vi "Draw Current Position Marker.vi"(8 "Error":errorcluster, 9 "Waveform":waveform(dbl), 10 "State":T1={"Measure ?"=[], "Direction"=[], "Loop ?"={"Start"=0, "Finish"=2}, "Storage Location"=[], "Show Current Location"=FALSE, "Current Location"=0, "Show y=0"=FALSE, "Program"=[], "Index"=0, "Average During Loop ?"=FALSE, "# of Loops"=1, "Loop Control"={0, 2}, "Units"="", "Digits"=0, "Significant Figures (F) or DP (T)"=FALSE, "Rate Mode"=FALSE, "Current Y value"=0.0, "Initial Value"=0.0} {"# of Loops" min=1 step=1; "Index" min=0 step=1; "Program"."Step" min=0.001 max=80.0 step=0.001 format="%.2f"; "Program"."Target" format="%.2f"}, 11 "Plots":cluster{"X":dbl[], "Y":dbl[]}[](array[cluster])) -> (0 "Error Out":errorcluster, 3 "Plots Out":cluster{"X":dbl[], "Y":dbl[]}[](array[cluster]))   [LabVIEW 2018, in "Multi Segment Waveform.xctl"]
doc: "Generates a waveform that is NaN apart from the one point at the given index position. The Y value of this point is the same as the corresponding point in the first waveform of the array input,"
uses:
  Multi Segment Waveform.xctl
  State.ctl
  <vilib>/Waveform/WDTOps.llb/WDT Get XY Value DBL.vi
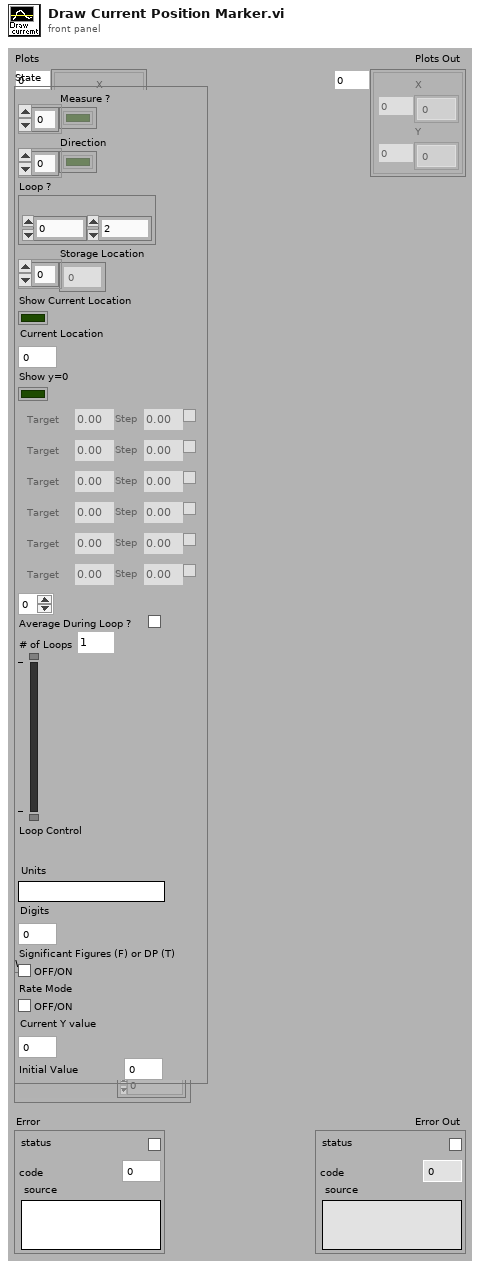
[diagram p1: front panel]
types:
  T1 = typedef "Multi Segment Waveform.xctl/State.ctl" = cluster{"Measure ?":bool[], "Direction":bool[], "Loop ?":cluster{"Start":i32, "Finish":i32}, "Storage Location":i32[], "Show Current Location":bool, "Current Location":i32, "Show y=0":bool, "Program":cluster{"Target":dbl, "Step":dbl, "Measure ?":bool}[], "Index":i32, "Average During Loop ?":bool, "# of Loops":u32, "Loop Control":cluster{i32, i32}, "Units":string, "Digits":i32, "Significant Figures (F) or DP (T)":bool, "Rate Mode":bool, "Current Y value":dbl, "Initial Value":dbl}
  T2 = cluster{"Target":dbl, "Step":dbl, "Measure ?":bool}[]
  T3 = cluster{"Target":dbl, "Step":dbl, "Measure ?":bool}
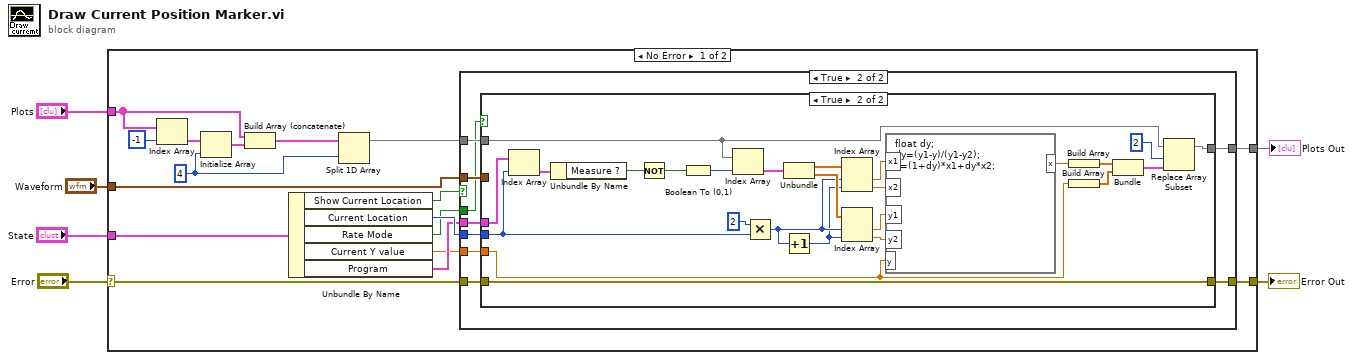
[diagram p0: block diagram]
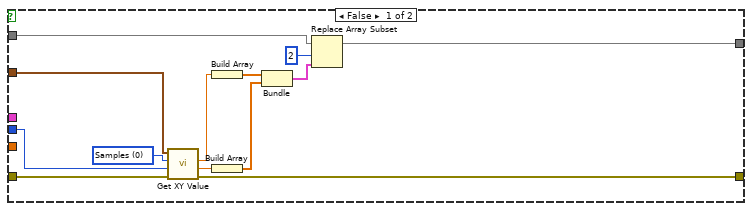
[diagram p3: hidden frame]
diagram:
  n1 = case shown="No Error" "Error" {
    selector: "Error" -> [w18 w74]
    tunnel: "Plots" -> [w13 w73]
    tunnel: "State" -> [w23 _]
    tunnel: "Waveform" -> [w21 _]
    tunnel: [w19 w73] -> w3
    tunnel: [w17 w74] -> w1
    frame No Error {
      w11 = 4 ("dimension size")
      n2 = Index Array(array=w13, index=-1) -> (element=w15:cluster{"X":dbl[], "Y":dbl[]})
      n3 = Initialize Array(w15, w11) -> (w14:cluster{"X":dbl[], "Y":dbl[]}[])
      n4 = Build Array (concatenate)(w13, w14) -> (w12:cluster{"X":dbl[], "Y":dbl[]}[])
      n5 = Unbundle By Name(w23) -> ("Show Current Location"=w22:bool, "Current Location"=w20:i32, "Rate Mode"=w9:bool, "Current Y value"=w7:dbl, "Program"=w8:T2)
      n6 = Split 1D Array(array=w12, index=w11) -> (first subarray=w10:cluster{"X":dbl[], "Y":dbl[]}[])  [unwired: 1 out]
      n7 = case shown="True" w22 {
        tunnel: w10 -> [w25 w32]
        tunnel: w21 -> [_ w34]
        tunnel: w20 -> [_ w33]
        tunnel: [w25 w31] -> w19
        tunnel: w18 -> [w24 w30]
        tunnel: [w24 w29] -> w17
        tunnel: w9 -> [_ w28]
        tunnel: w8 -> [_ w27]
        tunnel: w7 -> [_ w26]
        frame False {
        }
        frame True {
          n8 = case shown="True" w28 {
            tunnel: w34 -> [w46 _]
            tunnel: w33 -> [w45 w68]
            tunnel: w32 -> [w40 w50]
            tunnel: [w37 w49] -> w31
            tunnel: w30 -> [w36 w48]
            tunnel: [w35 w48] -> w29
            tunnel: w27 -> [_ w69]
            tunnel: w26 -> [_ w51]
            frame False {
              w47 = u16 0 items=["Samples", "Relative Time"] ("Y position format")
              n9 = call-poly <vilib>:"Get XY Value.vi"("error in (no error)"=w36, "Y position"=w45, "Y position format"=w47, "waveform in"=w46) -> ("error out"=w35:errorcluster, "Y value"=w43:dbl, "actual Y position"=w44:dbl)  [unwired: 5 out]
              n10 = Build Array(w44) -> (w42:dbl[])
              n11 = Build Array(w43) -> (w41:dbl[])
              n12 = Bundle(w42, w41) -> (w38:cluster{dbl[], dbl[]})  [unwired: 1 out]
              n13 = Replace Array Subset(array=w40, new element=w38, index=2) -> (w37:cluster{"X":dbl[], "Y":dbl[]}[])
            }
            frame True {
              n14 = Index Array(array=w69, index=w68) -> (element=w67:T3)
              n15 = Unbundle By Name(w67) -> ("Measure ?"=w66:bool)
              n16 = Not(x=w66) -> (.not. x?=w65:bool)
              n17 = Boolean To (0,1)(Boolean=w65) -> (0, 1=w64:i16)
              n18 = Index Array(array=w50, index=w64) -> (element=w72:cluster{"X":dbl[], "Y":dbl[]})
              n19 = Multiply(x=2, y=w68) -> (x*y=w62:i32)
              n20 = Unbundle(w72) -> ("X"=w63:dbl[], "Y"=w71:dbl[])
              n21 = Increment(x=w62) -> (x+1=w61:i32)
              n22 = Index Array(array=w63, index #1=w62, index #2=w61) -> (element #1=w60:dbl, element #2=w59:dbl)
              n23 = Index Array(array=w71, index #1=w62, index #2=w61) -> (element #1=w58:dbl, element #2=w57:dbl)
              n24 = formula code="float dy;\ndy=(y1-y)/(y1-y2);\nx=(1+dy)*x1+dy*x2;"("x1"=w60, "x2"=w59, "y1"=w58, "y2"=w57, "y"=w51) -> ("x"=w52:dbl)
              n25 = Build Array(w52) -> (w56:dbl[])
              n26 = Build Array(w51) -> (w55:dbl[])
              n27 = Bundle(w56, w55) -> (w53:cluster{dbl[], dbl[]})  [unwired: 1 out]
              n28 = Replace Array Subset(array=w50, new element=w53, index=2) -> (w49:cluster{"X":dbl[], "Y":dbl[]}[])
            }
          }
        }
      }
    }
    frame Error {
    }
  }
  "Plots Out" <- w3
  "Error Out" <- w1
